vi "App - analyze RUS V6.vi"() -> ()   [LabVIEW 2021] (continued)
"last mod"=timestamp(3493848079 s since 1904-01-01), "file name str"="D:\\Data\\Ultrasound\\LSCO\\LSCO22__130814c\\5_Cooling_2nd_try\\September_2014\\091714\\14.95900K_500_2500_2.10000V_0.00000T_Sep17-2014__21-21-19_001_091714.bin", "mod time(min)"=58230801.31666667, "file format"=enum."binary", "power(V)"=2.1, "Magn Field(T) "=0.0}, {"temperature"=14.952, "temperature str"="14.95200", "file path"=path "D:/Data/Ultrasound/LSCO/LSCO22__130814c/5_Cooling_2nd_try/September_2014/091714/14.95200K_500_2500_2.10000V_0.00000T_Sep17-2014__21-22-38_001_091714.bin", "last mod"=timestamp(3493848158 s since 1904-01-01), "file name str"="D:\\Data\\Ultrasound\\LSCO\\LSCO22__130814c\\5_Cooling_2nd_try\\September_2014\\091714\\14.95200K_500_2500_2.10000V_0.00000T_Sep17-2014__21-22-38_001_091714.bin", "mod time(min)"=58230802.63333333, "file format"=enum."binary", "power(V)"=2.1, "Magn Field(T) "=0.0}, {"temperature"=14.954, "temperature str"="14.95400", "file path"=path "D:/Data/Ultrasound/LSCO/LSCO22__130814c/5_Cooling_2nd_try/September_2014/091714/14.95400K_500_2500_2.10000V_0.00000T_Sep17-2014__21-23-58_001_091714.bin", "last mod"=timestamp(3493848238 s since 1904-01-01), "file name str"="D:\\Data\\Ultrasound\\LSCO\\LSCO22__130814c\\5_Cooling_2nd_try\\September_2014\\091714\\14.95400K_500_2500_2.10000V_0.00000T_Sep17-2014__21-23-58_001_091714.bin", "mod time(min)"=58230803.96666667, "file format"=enum."binary", "power(V)"=2.1, "Magn Field(T) "=0.0}, {"temperature"=14.948, "temperature str"="14.94800", "file path"=path "D:/Data/Ultrasound/LSCO/LSCO22__130814c/5_Cooling_2nd_try/September_2014/091714/14.94800K_500_2500_2.10000V_0.00000T_Sep17-2014__21-25-17_001_091714.bin", "last mod"=timestamp(3493848317 s since 1904-01-01), "file name str"="D:\\Data\\Ultrasound\\LSCO\\LSCO22__130814c\\5_Cooling_2nd_try\\September_2014\\091714\\14.94800K_500_2500_2.10000V_0.00000T_Sep17-2014__21-25-17_001_091714.bin", "mod time(min)"=58230805.28333333, "file format"=enum."binary", "power(V)"=2.1, "Magn Field(T) "=0.0}, {"temperature"=14.938, "temperature str"="14.93800", "file path"=path "D:/Data/Ultrasound/LSCO/LSCO22__130814c/5_Cooling_2nd_try/September_2014/091714/14.93800K_500_2500_2.10000V_0.00000T_Sep17-2014__21-26-37_001_091714.bin", "last mod"=timestamp(3493848397 s since 1904-01-01), "file name str"="D:\\Data\\Ultrasound\\LSCO\\LSCO22__130814c\\5_Cooling_2nd_try\\September_2014\\091714\\14.93800K_500_2500_2.10000V_0.00000T_Sep17-2014__21-26-37_001_091714.bin", "mod time(min)"=58230806.61666667, "file format"=enum."binary", "power(V)"=2.1, "Magn Field(T) "=0.0}, {"temperature"=14.942, "temperature str"="14.94200", "file path"=path "D:/Data/Ultrasound/LSCO/LSCO22__130814c/5_Cooling_2nd_try/September_2014/091714/14.94200K_500_2500_2.10000V_0.00000T_Sep17-2014__21-27-56_001_091714.bin", "last mod"=timestamp(3493848476 s since 1904-01-01), "file name str"="D:\\Data\\Ultrasound\\LSCO\\LSCO22__130814c\\5_Cooling_2nd_try\\September_2014\\091714\\14.94200K_500_2500_2.10000V_0.00000T_Sep17-2014__21-27-56_001_091714.bin", "mod time(min)"=58230807.93333333, "file format"=enum."binary", "power(V)"=2.1, "Magn Field(T) "=0.0}, {"temperature"=14.929, "temperature str"="14.92900", "file path"=path "D:/Data/Ultrasound/LSCO/LSCO22__130814c/5_Cooling_2nd_try/September_2014/091714/14.92900K_500_2500_2.10000V_0.00000T_Sep17-2014__21-29-15_001_091714.bin", "last mod"=timestamp(3493848555 s since 1904-01-01), "file name str"="D:\\Data\\Ultrasound\\LSCO\\LSCO22__130814c\\5_Cooling_2nd_try\\September_2014\\091714\\14.92900K_500_2500_2.10000V_0.00000T_Sep17-2014__21-29-15_001_091714.bin", "mod time(min)"=58230809.25, "file format"=enum."binary", "power(V)"=2.1, "Magn Field(T) "=0.0}, {"temperature"=14.927, "temperature str"="14.92700", "file path"=path "D:/Data/Ultrasound/LSCO/LSCO22__130814c/5_Cooling_2nd_try/September_2014/091714/14.92700K_500_2500_2.10000V_0.00000T_Sep17-2014__21-30-35_001_091714.bin", "last mod"=timestamp(3493848635 s since 1904-01-01), "file name str"="D:\\Data\\Ultrasound\\LSCO\\LSCO22__130814c\\5_Cooling_2nd_try\\September_2014\\091714\\14.92700K_500_2500_2.10000V_0.00000T_Sep17-2014__21-30-35_001_091714.bin", "mod time(min)"=58230810.583333336, "file format"=enum."binary", "power(V)"=2.1, "Magn Field(T) "=0.0}, {"temperature"=14.922, "temperature str"="14.92200", "file path"=path "D:/Data/Ultrasound/LSCO/LSCO22__130814c/5_Cooling_2nd_try/September_2014/091714/14.92200K_500_2500_2.10000V_0.00000T_Sep17-2014__21-31-54_001_091714.bin", "last mod"=timestamp(3493848714 s since 1904-01-01), "file name str"="D:\\Data\\Ultrasound\\LSCO\\LSCO22__130814c\\5_Cooling_2nd_try\\September_2014\\091714\\14.92200K_500_2500_2.10000V_0.00000T_Sep17-2014__21-31-54_001_091714.bin", "mod time(min)"=58230811.9, "file format"=enum."binary", "power(V)"=2.1, "Magn Field(T) "=0.0}, {"temperature"=14.929, "temperature str"="14.92900", "file path"=path "D:/Data/Ultrasound/LSCO/LSCO22__130814c/5_Cooling_2nd_try/September_2014/091714/14.92900K_500_2500_2.10000V_0.00000T_Sep17-2014__21-33-14_001_091714.bin", "last mod"=timestamp(3493848794 s since 1904-01-01), "file name str"="D:\\Data\\Ultrasound\\LSCO\\LSCO22__130814c\\5_Cooling_2nd_try\\September_2014\\091714\\14.92900K_500_2500_2.10000V_0.00000T_Sep17-2014__21-33-14_001_091714.bin", "mod time(min)"=58230813.233333334, "file format"=enum."binary", "power(V)"=2.1, "Magn Field(T) "=0.0}, {"temperature"=14.927, "temperature str"="14.92700", "file path"=path "D:/Data/Ultrasound/LSCO/LSCO22__130814c/5_Cooling_2nd_try/September_2014/091714/14.92700K_500_2500_2.10000V_0.00000T_Sep17-2014__21-34-33_001_091714.bin", "last mod"=timestamp(3493848873 s since 1904-01-01), "file name str"="D:\\Data\\Ultrasound\\LSCO\\LSCO22__130814c\\5_Cooling_2nd_try\\September_2014\\091714\\14.92700K_500_2500_2.10000V_0.00000T_Sep17-2014__21-34-33_001_091714.bin", "mod time(min)"=58230814.55, "file format"=enum."binary", "power(V)"=2.1, "Magn Field(T) "=0.0}, {"temperature"=14.926, "temperature str"="14.92600", "file path"=path "D:/Data/Ultrasound/LSCO/LSCO22__130814c/5_Cooling_2nd_try/September_2014/091714/14.92600K_500_2500_2.10000V_0.00000T_Sep17-2014__21-35-52_001_091714.bin", "last mod"=timestamp(3493848952 s since 1904-01-01), "file name str"="D:\\Data\\Ultrasound\\LSCO\\LSCO22__130814c\\5_Cooling_2nd_try\\September_2014\\091714\\14.92600K_500_2500_2.10000V_0.00000T_Sep17-2014__21-35-52_001_091714.bin", "mod time(min)"=58230815.86666667, "file format"=enum."binary", "power(V)"=2.1, "Magn Field(T) "=0.0}, {"temperature"=14.912, "temperature str"="14.91200", "file path"=path "D:/Data/Ultrasound/LSCO/LSCO22__130814c/5_Cooling_2nd_try/September_2014/091714/14.91200K_500_2500_2.10000V_0.00000T_Sep17-2014__21-37-12_001_091714.bin", "last mod"=timestamp(3493849032 s since 1904-01-01), "file name str"="D:\\Data\\Ultrasound\\LSCO\\LSCO22__130814c\\5_Cooling_2nd_try\\September_2014\\091714\\14.91200K_500_2500_2.10000V_0.00000T_Sep17-2014__21-37-12_001_091714.bin", "mod time(min)"=58230817.2, "file format"=enum."binary", "power(V)"=2.1, "Magn Field(T) "=0.0}, {"temperature"=14.915, "temperature str"="14.91500", "file path"=path "D:/Data/Ultrasound/LSCO/LSCO22__130814c/5_Cooling_2nd_try/September_2014/091714/14.91500K_500_2500_2.10000V_0.00000T_Sep17-2014__21-38-31_001_091714.bin", "last mod"=timestamp(3493849111 s since 1904-01-01), "file name str"="D:\\Data\\Ultrasound\\LSCO\\LSCO22__130814c\\5_Cooling_2nd_try\\September_2014\\091714\\14.91500K_500_2500_2.10000V_0.00000T_Sep17-2014__21-38-31_001_091714.bin", "mod time(min)"=58230818.516666666, "file format"=enum."binary", "power(V)"=2.1, "Magn Field(T) "=0.0}, {"temperature"=14.912, "temperature str"="14.91200", "file path"=path "D:/Data/Ultrasound/LSCO/LSCO22__130814c/5_Cooling_2nd_try/September_2014/091714/14.91200K_500_2500_2.10000V_0.00000T_Sep17-2014__21-39-50_001_091714.bin", "last mod"=timestamp(3493849190 s since 1904-01-01), "file name str"="D:\\Data\\Ultrasound\\LSCO\\LSCO22__130814c\\5_Cooling_2nd_try\\September_2014\\091714\\14.91200K_500_2500_2.10000V_0.00000T_Sep17-2014__21-39-50_001_091714.bin", "mod time(min)"=58230819.833333336, "file format"=enum."binary", "power(V)"=2.1, "Magn Field(T) "=0.0}, {"temperature"=14.91, "temperature str"="14.91000", "file path"=path "D:/Data/Ultrasound/LSCO/LSCO22__130814c/5_Cooling_2nd_try/September_2014/091714/14.91000K_500_2500_2.10000V_0.00000T_Sep17-2014__21-41-10_001_091714.bin", "last mod"=timestamp(3493849270 s since 1904-01-01), "file name str"="D:\\Data\\Ultrasound\\LSCO\\LSCO22__130814c\\5_Cooling_2nd_try\\September_2014\\091714\\14.91000K_500_2500_2.10000V_0.00000T_Sep17-2014__21-41-10_001_091714.bin", "mod time(min)"=58230821.166666664, "file format"=enum."binary", "power(V)"=2.1, "Magn Field(T) "=0.0}, {"temperature"=14.907, "temperature str"="14.90700", "file path"=path "D:/Data/Ultrasound/LSCO/LSCO22__130814c/5_Cooling_2nd_try/September_2014/091714/14.90700K_500_2500_2.10000V_0.00000T_Sep17-2014__21-42-29_001_091714.bin", "last mod"=timestamp(3493849349 s since 1904-01-01), "file name str"="D:\\Data\\Ultrasound\\LSCO\\LSCO22__130814c\\5_Cooling_2nd_try\\September_2014\\091714\\14.90700K_500_2500_2.10000V_0.00000T_Sep17-2014__21-42-29_001_091714.bin", "mod time(min)"=58230822.483333334, "file format"=enum."binary", "power(V)"=2.1, "Magn Field(T) "=0.0}, {"temperature"=14.908, "temperature str"="14.90800", "file path"=path "D:/Data/Ultrasound/LSCO/LSCO22__130814c/5_Cooling_2nd_try/September_2014/091714/14.90800K_500_2500_2.10000V_0.00000T_Sep17-2014__21-43-49_001_091714.bin", "last mod"=timestamp(3493849429 s since 1904-01-01), "file name str"="D:\\Data\\Ultrasound\\LSCO\\LSCO22__130814c\\5_Cooling_2nd_try\\September_2014\\091714\\14.90800K_500_2500_2.10000V_0.00000T_Sep17-2014__21-43-49_001_091714.bin", "mod time(min)"=58230823.81666667, "file format"=enum."binary", "power(V)"=2.1, "Magn Field(T) "=0.0}, {"temperature"=14.9, "temperature str"="14.90000", "file path"=path "D:/Data/Ultrasound/LSCO/LSCO22__130814c/5_Cooling_2nd_try/September_2014/091714/14.90000K_500_2500_2.10000V_0.00000T_Sep17-2014__21-45-08_001_091714.bin", "last mod"=timestamp(3493849508 s since 1904-01-01), "file name str"="D:\\Data\\Ultrasound\\LSCO\\LSCO22__130814c\\5_Cooling_2nd_try\\September_2014\\091714\\14.90000K_500_2500_2.10000V_0.00000T_Sep17-2014__21-45-08_001_091714.bin", "mod time(min)"=58230825.13333333, "file format"=enum."binary", "power(V)"=2.1, "Magn Field(T) "=0.0}, {"temperature"=14.9, "temperature str"="14.90000", "file path"=path "D:/Data/Ultrasound/LSCO/LSCO22__130814c/5_Cooling_2nd_try/September_2014/091714/14.90000K_500_2500_2.10000V_0.00000T_Sep17-2014__21-46-27_001_091714.bin", "last mod"=timestamp(3493849587 s since 1904-01-01), "file name str"="D:\\Data\\Ultrasound\\LSCO\\LSCO22__130814c\\5_Cooling_2nd_try\\September_2014\\091714\\14.90000K_500_2500_2.10000V_0.00000T_Sep17-2014__21-46-27_001_091714.bin", "mod time(min)"=58230826.45, "file format"=enum."binary", "power(V)"=2.1, "Magn Field(T) "=0.0}, {"temperature"=14.895, "temperature str"="14.89500", "file path"=path "D:/Data/Ultrasound/LSCO/LSCO22__130814c/5_Cooling_2nd_try/September_2014/091714/14.89500K_500_2500_2.10000V_0.00000T_Sep17-2014__21-47-47_001_091714.bin", "last mod"=timestamp(3493849667 s since 1904-01-01), "file name str"="D:\\Data\\Ultrasound\\LSCO\\LSCO22__130814c\\5_Cooling_2nd_try\\September_2014\\091714\\14.89500K_500_2500_2.10000V_0.00000T_Sep17-2014__21-47-47_001_091714.bin", "mod time(min)"=58230827.78333333, "file format"=enum."binary", "power(V)"=2.1, "Magn Field(T) "=0.0}, {"temperature"=14.89, "temperature str"="14.89000", "file path"=path "D:/Data/Ultrasound/LSCO/LSCO22__130814c/5_Cooling_2nd_try/September_2014/091714/14.89000K_500_2500_2.10000V_0.00000T_Sep17-2014__21-49-06_001_091714.bin", "last mod"=timestamp(3493849746 s since 1904-01-01), "file name str"="D:\\Data\\Ultrasound\\LSCO\\LSCO22__130814c\\5_Cooling_2nd_try\\September_2014\\091714\\14.89000K_500_2500_2.10000V_0.00000T_Sep17-2014__21-49-06_001_091714.bin", "mod time(min)"=58230829.1, "file format"=enum."binary", "power(V)"=2.1, "Magn Field(T) "=0.0}, {"temperature"=14.886, "temperature str"="14.88600", "file path"=path "D:/Data/Ultrasound/LSCO/LSCO22__130814c/5_Cooling_2nd_try/September_2014/091714/14.88600K_500_2500_2.10000V_0.00000T_Sep17-2014__21-50-26_001_091714.bin", "last mod"=timestamp(3493849826 s since 1904-01-01), "file name str"="D:\\Data\\Ultrasound\\LSCO\\LSCO22__130814c\\5_Cooling_2nd_try\\September_2014\\091714\\14.88600K_500_2500_2.10000V_0.00000T_Sep17-2014__21-50-26_001_091714.bin", "mod time(min)"=58230830.43333333, "file format"=enum."binary", "power(V)"=2.1, "Magn Field(T) "=0.0}, {"temperature"=14.883, "temperature str"="14.88300", "file path"=path "D:/Data/Ultrasound/LSCO/LSCO22__130814c/5_Cooling_2nd_try/September_2014/091714/14.88300K_500_2500_2.10000V_0.00000T_Sep17-2014__21-51-45_001_091714.bin", "last mod"=timestamp(3493849905 s since 1904-01-01), "file name str"="D:\\Data\\Ultrasound\\LSCO\\LSCO22__130814c\\5_Cooling_2nd_try\\September_2014\\091714\\14.88300K_500_2500_2.10000V_0.00000T_Sep17-2014__21-51-45_001_091714.bin", "mod time(min)"=58230831.75, "file format"=enum."binary", "power(V)"=2.1, "Magn Field(T) "=0.0}, {"temperature"=14.876, "temperature str"="14.87600", "file path"=path "D:/Data/Ultrasound/LSCO/LSCO22__130814c/5_Cooling_2nd_try/September_2014/091714/14.87600K_500_2500_2.10000V_0.00000T_Sep17-2014__21-53-04_001_091714.bin", "last mod"=timestamp(3493849984 s since 1904-01-01), "file name str"="D:\\Data\\Ultrasound\\LSCO\\LSCO22__130814c\\5_Cooling_2nd_try\\September_2014\\091714\\14.87600K_500_2500_2.10000V_0.00000T_Sep17-2014__21-53-04_001_091714.bin", "mod time(min)"=58230833.06666667, "file format"=enum."binary", "power(V)"=2.1, "Magn Field(T) "=0.0}, {"temperature"=14.875, "temperature str"="14.87500", "file path"=path "D:/Data/Ultrasound/LSCO/LSCO22__130814c/5_Cooling_2nd_try/September_2014/091714/14.87500K_500_2500_2.10000V_0.00000T_Sep17-2014__21-54-24_001_091714.bin", "last mod"=timestamp(3493850064 s since 1904-01-01), "file name str"="D:\\Data\\Ultrasound\\LSCO\\LSCO22__130814c\\5_Cooling_2nd_try\\September_2014\\091714\\14.87500K_500_2500_2.10000V_0.00000T_Sep17-2014__21-54-24_001_091714.bin", "mod time(min)"=58230834.4, "file format"=enum."binary", "power(V)"=2.1, "Magn Field(T) "=0.0}, {"temperature"=14.872, "temperature str"="14.87200", "file path"=path "D:/Data/Ultrasound/LSCO/LSCO22__130814c/5_Cooling_2nd_try/September_2014/091714/14.87200K_500_2500_2.10000V_0.00000T_Sep17-2014__21-55-43_001_091714.bin", "last mod"=timestamp(3493850143 s since 1904-01-01), "file name str"="D:\\Data\\Ultrasound\\LSCO\\LSCO22__130814c\\5_Cooling_2nd_try\\September_2014\\091714\\14.87200K_500_2500_2.10000V_0.00000T_Sep17-2014__21-55-43_001_091714.bin", "mod time(min)"=58230835.71666667, "file format"=enum."binary", "power(V)"=2.1, "Magn Field(T) "=0.0}, {"temperature"=14.874, "temperature str"="14.87400", "file path"=path "D:/Data/Ultrasound/LSCO/LSCO22__130814c/5_Cooling_2nd_try/September_2014/091714/14.87400K_500_2500_2.10000V_0.00000T_Sep17-2014__21-57-02_001_091714.bin", "last mod"=timestamp(3493850222 s since 1904-01-01), "file name str"="D:\\Data\\Ultrasound\\LSCO\\LSCO22__130814c\\5_Cooling_2nd_try\\September_2014\\091714\\14.87400K_500_2500_2.10000V_0.00000T_Sep17-2014__21-57-02_001_091714.bin", "mod time(min)"=58230837.03333333, "file format"=enum."binary", "power(V)"=2.1, "Magn Field(T) "=0.0}, {"temperature"=14.877, "temperature str"="14.87700", "file path"=path "D:/Data/Ultrasound/LSCO/LSCO22__130814c/5_Cooling_2nd_try/September_2014/091714/14.87700K_500_2500_2.10000V_0.00000T_Sep17-2014__21-58-22_001_091714.bin", "last mod"=timestamp(3493850302 s since 1904-01-01), "file name str"="D:\\Data\\Ultrasound\\LSCO\\LSCO22__130814c\\5_Cooling_2nd_try\\September_2014\\091714\\14.87700K_500_2500_2.10000V_0.00000T_Sep17-2014__21-58-22_001_091714.bin", "mod time(min)"=58230838.36666667, "file format"=enum."binary", "power(V)"=2.1, "Magn Field(T) "=0.0}, {"temperature"=14.872, "temperature str"="14.87200", "file path"=path "D:/Data/Ultrasound/LSCO/LSCO22__130814c/5_Cooling_2nd_try/September_2014/091714/14.87200K_500_2500_2.10000V_0.00000T_Sep17-2014__21-59-41_001_091714.bin", "last mod"=timestamp(3493850381 s since 1904-01-01), "file name str"="D:\\Data\\Ultrasound\\LSCO\\LSCO22__130814c\\5_Cooling_2nd_try\\September_2014\\091714\\14.87200K_500_2500_2.10000V_0.00000T_Sep17-2014__21-59-41_001_091714.bin", "mod time(min)"=58230839.68333333, "file format"=enum."binary", "power(V)"=2.1, "Magn Field(T) "=0.0}, {"temperature"=14.873, "temperature str"="14.87300", "file path"=path "D:/Data/Ultrasound/LSCO/LSCO22__130814c/5_Cooling_2nd_try/September_2014/091714/14.87300K_500_2500_2.10000V_0.00000T_Sep17-2014__22-01-01_001_091714.bin", "last mod"=timestamp(3493850461 s since 1904-01-01), "file name str"="D:\\Data\\Ultrasound\\LSCO\\LSCO22__130814c\\5_Cooling_2nd_try\\September_2014\\091714\\14.87300K_500_2500_2.10000V_0.00000T_Sep17-2014__22-01-01_001_091714.bin", "mod time(min)"=58230841.016666666, "file format"=enum."binary", "power(V)"=2.1, "Magn Field(T) "=0.0}, {"temperature"=14.873, "temperature str"="14.87300", "file path"=path "D:/Data/Ultrasound/LSCO/LSCO22__130814c/5_Cooling_2nd_try/September_2014/091714/14.87300K_500_2500_2.10000V_0.00000T_Sep17-2014__22-02-20_001_091714.bin", "last mod"=timestamp(3493850540 s since 1904-01-01), "file name str"="D:\\Data\\Ultrasound\\LSCO\\LSCO22__130814c\\5_Cooling_2nd_try\\September_2014\\091714\\14.87300K_500_2500_2.10000V_0.00000T_Sep17-2014__22-02-20_001_091714.bin", "mod time(min)"=58230842.333333336, "file format"=enum."binary", "power(V)"=2.1, "Magn Field(T) "=0.0}, {"temperature"=14.868, "temperature str"="14.86800", "file path"=path "D:/Data/Ultrasound/LSCO/LSCO22__130814c/5_Cooling_2nd_try/September_2014/091714/14.86800K_500_2500_2.10000V_0.00000T_Sep17-2014__22-03-39_001_091714.bin", "last mod"=timestamp(3493850619 s since 1904-01-01), "file name str"="D:\\Data\\Ultrasound\\LSCO\\LSCO22__130814c\\5_Cooling_2nd_try\\September_2014\\091714\\14.86800K_500_2500_2.10000V_0.00000T_Sep17-2014__22-03-39_001_091714.bin", "mod time(min)"=58230843.65, "file format"=enum."binary", "power(V)"=2.1, "Magn Field(T) "=0.0}, {"temperature"=14.859, "temperature str"="14.85900", "file path"=path "D:/Data/Ultrasound/LSCO/LSCO22__130814c/5_Cooling_2nd_try/September_2014/091714/14.85900K_500_2500_2.10000V_0.00000T_Sep17-2014__22-04-59_001_091714.bin", "last mod"=timestamp(3493850699 s since 1904-01-01), "file name str"="D:\\Data\\Ultrasound\\LSCO\\LSCO22__130814c\\5_Cooling_2nd_try\\September_2014\\091714\\14.85900K_500_2500_2.10000V_0.00000T_Sep17-2014__22-04-59_001_091714.bin", "mod time(min)"=58230844.983333334, "file format"=enum."binary", "power(V)"=2.1, "Magn Field(T) "=0.0}, {"temperature"=14.866, "temperature str"="14.86600", "file path"=path "D:/Data/Ultrasound/LSCO/LSCO22__130814c/5_Cooling_2nd_try/September_2014/091714/14.86600K_500_2500_2.10000V_0.00000T_Sep17-2014__22-06-18_001_091714.bin", "last mod"=timestamp(3493850778 s since 1904-01-01), "file name str"="D:\\Data\\Ultrasound\\LSCO\\LSCO22__130814c\\5_Cooling_2nd_try\\September_2014\\091714\\14.86600K_500_2500_2.10000V_0.00000T_Sep17-2014__22-06-18_001_091714.bin", "mod time(min)"=58230846.3, "file format"=enum."binary", "power(V)"=2.1, "Magn Field(T) "=0.0}, {"temperature"=14.858, "temperature str"="14.85800", "file path"=path "D:/Data/Ultrasound/LSCO/LSCO22__130814c/5_Cooling_2nd_try/September_2014/091714/14.85800K_500_2500_2.10000V_0.00000T_Sep17-2014__22-07-37_001_091714.bin", "last mod"=timestamp(3493850857 s since 1904-01-01), "file name str"="D:\\Data\\Ultrasound\\LSCO\\LSCO22__130814c\\5_Cooling_2nd_try\\September_2014\\091714\\14.85800K_500_2500_2.10000V_0.00000T_Sep17-2014__22-07-37_001_091714.bin", "mod time(min)"=58230847.61666667, "file format"=enum."binary", "power(V)"=2.1, "Magn Field(T) "=0.0}, {"temperature"=14.86, "temperature str"="14.86000", "file path"=path "D:/Data/Ultrasound/LSCO/LSCO22__130814c/5_Cooling_2nd_try/September_2014/091714/14.86000K_500_2500_2.10000V_0.00000T_Sep17-2014__22-08-57_001_091714.bin", "last mod"=timestamp(3493850937 s since 1904-01-01), "file name str"="D:\\Data\\Ultrasound\\LSCO\\LSCO22__130814c\\5_Cooling_2nd_try\\September_2014\\091714\\14.86000K_500_2500_2.10000V_0.00000T_Sep17-2014__22-08-57_001_091714.bin", "mod time(min)"=58230848.95, "file format"=enum."binary", "power(V)"=2.1, "Magn Field(T) "=0.0}, {"temperature"=14.866, "temperature str"="14.86600", "file path"=path "D:/Data/Ultrasound/LSCO/LSCO22__130814c/5_Cooling_2nd_try/September_2014/091714/14.86600K_500_2500_2.10000V_0.00000T_Sep17-2014__22-10-16_001_091714.bin", "last mod"=timestamp(3493851016 s since 1904-01-01), "file name str"="D:\\Data\\Ultrasound\\LSCO\\LSCO22__130814c\\5_Cooling_2nd_try\\September_2014\\091714\\14.86600K_500_2500_2.10000V_0.00000T_Sep17-2014__22-10-16_001_091714.bin", "mod time(min)"=58230850.266666666, "file format"=enum."binary", "power(V)"=2.1, "Magn Field(T) "=0.0}, {"temperature"=14.857, "temperature str"="14.85700", "file path"=path "D:/Data/Ultrasound/LSCO/LSCO22__130814c/5_Cooling_2nd_try/September_2014/091714/14.85700K_500_2500_2.10000V_0.00000T_Sep17-2014__22-11-36_001_091714.bin", "last mod"=timestamp(3493851096 s since 1904-01-01), "file name str"="D:\\Data\\Ultrasound\\LSCO\\LSCO22__130814c\\5_Cooling_2nd_try\\September_2014\\091714\\14.85700K_500_2500_2.10000V_0.00000T_Sep17-2014__22-11-36_001_091714.bin", "mod time(min)"=58230851.6, "file format"=enum."binary", "power(V)"=2.1, "Magn Field(T) "=0.0}, {"temperature"=14.853, "temperature str"="14.85300", "file path"=path "D:/Data/Ultrasound/LSCO/LSCO22__130814c/5_Cooling_2nd_try/September_2014/091714/14.85300K_500_2500_2.10000V_0.00000T_Sep17-2014__22-12-55_001_091714.bin", "last mod"=timestamp(3493851175 s since 1904-01-01), "file name str"="D:\\Data\\Ultrasound\\LSCO\\LSCO22__130814c\\5_Cooling_2nd_try\\September_2014\\091714\\14.85300K_500_2500_2.10000V_0.00000T_Sep17-2014__22-12-55_001_091714.bin", "mod time(min)"=58230852.916666664, "file format"=enum."binary", "power(V)"=2.1, "Magn Field(T) "=0.0}, {"temperature"=14.852, "temperature str"="14.85200", "file path"=path "D:/Data/Ultrasound/LSCO/LSCO22__130814c/5_Cooling_2nd_try/September_2014/091714/14.85200K_500_2500_2.10000V_0.00000T_Sep17-2014__22-14-14_001_091714.bin", "last mod"=timestamp(3493851254 s since 1904-01-01), "file name str"="D:\\Data\\Ultrasound\\LSCO\\LSCO22__130814c\\5_Cooling_2nd_try\\September_2014\\091714\\14.85200K_500_2500_2.10000V_0.00000T_Sep17-2014__22-14-14_001_091714.bin", "mod time(min)"=58230854.233333334, "file format"=enum."binary", "power(V)"=2.1, "Magn Field(T) "=0.0}, {"temperature"=14.844, "temperature str"="14.84400", "file path"=path "D:/Data/Ultrasound/LSCO/LSCO22__130814c/5_Cooling_2nd_try/September_2014/091714/14.84400K_500_2500_2.10000V_0.00000T_Sep17-2014__22-15-34_001_091714.bin", "last mod"=timestamp(3493851334 s since 1904-01-01), "file name str"="D:\\Data\\Ultrasound\\LSCO\\LSCO22__130814c\\5_Cooling_2nd_try\\September_2014\\091714\\14.84400K_500_2500_2.10000V_0.00000T_Sep17-2014__22-15-34_001_091714.bin", "mod time(min)"=58230855.56666667, "file format"=enum."binary", "power(V)"=2.1, "Magn Field(T) "=0.0}, {"temperature"=14.841, "temperature str"="14.84100", "file path"=path "D:/Data/Ultrasound/LSCO/LSCO22__130814c/5_Cooling_2nd_try/September_2014/091714/14.84100K_500_2500_2.10000V_0.00000T_Sep17-2014__22-16-53_001_091714.bin", "last mod"=timestamp(3493851413 s since 1904-01-01), "file name str"="D:\\Data\\Ultrasound\\LSCO\\LSCO22__130814c\\5_Cooling_2nd_try\\September_2014\\091714\\14.84100K_500_2500_2.10000V_0.00000T_Sep17-2014__22-16-53_001_091714.bin", "mod time(min)"=58230856.88333333, "file format"=enum."binary", "power(V)"=2.1, "Magn Field(T) "=0.0}, {"temperature"=14.835, "temperature str"="14.83500", "file path"=path "D:/Data/Ultrasound/LSCO/LSCO22__130814c/5_Cooling_2nd_try/September_2014/091714/14.83500K_500_2500_2.10000V_0.00000T_Sep17-2014__22-18-12_001_091714.bin", "last mod"=timestamp(3493851492 s since 1904-01-01), "file name str"="D:\\Data\\Ultrasound\\LSCO\\LSCO22__130814c\\5_Cooling_2nd_try\\September_2014\\091714\\14.83500K_500_2500_2.10000V_0.00000T_Sep17-2014__22-18-12_001_091714.bin", "mod time(min)"=58230858.2, "file format"=enum."binary", "power(V)"=2.1, "Magn Field(T) "=0.0}, {"temperature"=14.822, "temperature str"="14.82200", "file path"=path "D:/Data/Ultrasound/LSCO/LSCO22__130814c/5_Cooling_2nd_try/September_2014/091714/14.82200K_500_2500_2.10000V_0.00000T_Sep17-2014__22-19-32_001_091714.bin", "last mod"=timestamp(3493851572 s since 1904-01-01), "file name str"="D:\\Data\\Ultrasound\\LSCO\\LSCO22__130814c\\5_Cooling_2nd_try\\September_2014\\091714\\14.82200K_500_2500_2.10000V_0.00000T_Sep17-2014__22-19-32_001_091714.bin", "mod time(min)"=58230859.53333333, "file format"=enum."binary", "power(V)"=2.1, "Magn Field(T) "=0.0}, {"temperature"=14.821, "temperature str"="14.82100", "file path"=path "D:/Data/Ultrasound/LSCO/LSCO22__130814c/5_Cooling_2nd_try/September_2014/091714/14.82100K_500_2500_2.10000V_0.00000T_Sep17-2014__22-20-51_001_091714.bin", "last mod"=timestamp(3493851651 s since 1904-01-01), "file name str"="D:\\Data\\Ultrasound\\LSCO\\LSCO22__130814c\\5_Cooling_2nd_try\\September_2014\\091714\\14.82100K_500_2500_2.10000V_0.00000T_Sep17-2014__22-20-51_001_091714.bin", "mod time(min)"=58230860.85, "file format"=enum."binary", "power(V)"=2.1, "Magn Field(T) "=0.0}, {"temperature"=14.824, "temperature str"="14.82400", "file path"=path "D:/Data/Ultrasound/LSCO/LSCO22__130814c/5_Cooling_2nd_try/September_2014/091714/14.82400K_500_2500_2.10000V_0.00000T_Sep17-2014__22-22-11_001_091714.bin", "last mod"=timestamp(3493851731 s since 1904-01-01), "file name str"="D:\\Data\\Ultrasound\\LSCO\\LSCO22__130814c\\5_Cooling_2nd_try\\September_2014\\091714\\14.82400K_500_2500_2.10000V_0.00000T_Sep17-2014__22-22-11_001_091714.bin", "mod time(min)"=58230862.18333333, "file format"=enum."binary", "power(V)"=2.1, "Magn Field(T) "=0.0}, {"temperature"=14.817, "temperature str"="14.81700", "file path"=path "D:/Data/Ultrasound/LSCO/LSCO22__130814c/5_Cooling_2nd_try/September_2014/091714/14.81700K_500_2500_2.10000V_0.00000T_Sep17-2014__22-23-30_001_091714.bin", "last mod"=timestamp(3493851810 s since 1904-01-01), "file name str"="D:\\Data\\Ultrasound\\LSCO\\LSCO22__130814c\\5_Cooling_2nd_try\\September_2014\\091714\\14.81700K_500_2500_2.10000V_0.00000T_Sep17-2014__22-23-30_001_091714.bin", "mod time(min)"=58230863.5, "file format"=enum."binary", "power(V)"=2.1, "Magn Field(T) "=0.0}, {"temperature"=14.811, "temperature str"="14.81100", "file path"=path "D:/Data/Ultrasound/LSCO/LSCO22__130814c/5_Cooling_2nd_try/September_2014/091714/14.81100K_500_2500_2.10000V_0.00000T_Sep17-2014__22-24-49_001_091714.bin", "last mod"=timestamp(3493851889 s since 1904-01-01), "file name str"="D:\\Data\\Ultrasound\\LSCO\\LSCO22__130814c\\5_Cooling_2nd_try\\September_2014\\091714\\14.81100K_500_2500_2.10000V_0.00000T_Sep17-2014__22-24-49_001_091714.bin", "mod time(min)"=58230864.81666667, "file format"=enum."binary", "power(V)"=2.1, "Magn Field(T) "=0.0}, {"temperature"=14.805, "temperature str"="14.80500", "file path"=path "D:/Data/Ultrasound/LSCO/LSCO22__130814c/5_Cooling_2nd_try/September_2014/091714/14.80500K_500_2500_2.10000V_0.00000T_Sep17-2014__22-26-09_001_091714.bin", "last mod"=timestamp(3493851969 s since 1904-01-01), "file name str"="D:\\Data\\Ultrasound\\LSCO\\LSCO22__130814c\\5_Cooling_2nd_try\\September_2014\\091714\\14.80500K_500_2500_2.10000V_0.00000T_Sep17-2014__22-26-09_001_091714.bin", "mod time(min)"=58230866.15, "file format"=enum."binary", "power(V)"=2.1, "Magn Field(T) "=0.0}, {"temperature"=14.791, "temperature str"="14.79100", "file path"=path "D:/Data/Ultrasound/LSCO/LSCO22__130814c/5_Cooling_2nd_try/September_2014/091714/14.79100K_500_2500_2.10000V_0.00000T_Sep17-2014__22-27-28_001_091714.bin", "last mod"=timestamp(3493852048 s since 1904-01-01), "file name str"="D:\\Data\\Ultrasound\\LSCO\\LSCO22__130814c\\5_Cooling_2nd_try\\September_2014\\091714\\14.79100K_500_2500_2.10000V_0.00000T_Sep17-2014__22-27-28_001_091714.bin", "mod time(min)"=58230867.46666667, "file format"=enum."binary", "power(V)"=2.1, "Magn Field(T) "=0.0}, {"temperature"=14.787, "temperature str"="14.78700", "file path"=path "D:/Data/Ultrasound/LSCO/LSCO22__130814c/5_Cooling_2nd_try/September_2014/091714/14.78700K_500_2500_2.10000V_0.00000T_Sep17-2014__22-28-48_001_091714.bin", "last mod"=timestamp(3493852128 s since 1904-01-01), "file name str"="D:\\Data\\Ultrasound\\LSCO\\LSCO22__130814c\\5_Cooling_2nd_try\\September_2014\\091714\\14.78700K_500_2500_2.10000V_0.00000T_Sep17-2014__22-28-48_001_091714.bin", "mod time(min)"=58230868.8, "file format"=enum."binary", "power(V)"=2.1, "Magn Field(T) "=0.0}, {"temperature"=14.778, "temperature str"="14.77800", "file path"=path "D:/Data/Ultrasound/LSCO/LSCO22__130814c/5_Cooling_2nd_try/September_2014/091714/14.77800K_500_2500_2.10000V_0.00000T_Sep17-2014__22-30-07_001_091714.bin", "last mod"=timestamp(3493852207 s since 1904-01-01), "file name str"="D:\\Data\\Ultrasound\\LSCO\\LSCO22__130814c\\5_Cooling_2nd_try\\September_2014\\091714\\14.77800K_500_2500_2.10000V_0.00000T_Sep17-2014__22-30-07_001_091714.bin", "mod time(min)"=58230870.11666667, "file format"=enum."binary", "power(V)"=2.1, "Magn Field(T) "=0.0}, {"temperature"=14.773, "temperature str"="14.77300", "file path"=path "D:/Data/Ultrasound/LSCO/LSCO22__130814c/5_Cooling_2nd_try/September_2014/091714/14.77300K_500_2500_2.10000V_0.00000T_Sep17-2014__22-31-26_001_091714.bin", "last mod"=timestamp(3493852286 s since 1904-01-01), "file name str"="D:\\Data\\Ultrasound\\LSCO\\LSCO22__130814c\\5_Cooling_2nd_try\\September_2014\\091714\\14.77300K_500_2500_2.10000V_0.00000T_Sep17-2014__22-31-26_001_091714.bin", "mod time(min)"=58230871.43333333, "file format"=enum."binary", "power(V)"=2.1, "Magn Field(T) "=0.0}, {"temperature"=14.769, "temperature str"="14.76900", "file path"=path "D:/Data/Ultrasound/LSCO/LSCO22__130814c/5_Cooling_2nd_try/September_2014/091714/14.76900K_500_2500_2.10000V_0.00000T_Sep17-2014__22-32-46_001_091714.bin", "last mod"=timestamp(3493852366 s since 1904-01-01), "file name str"="D:\\Data\\Ultrasound\\LSCO\\LSCO22__130814c\\5_Cooling_2nd_try\\September_2014\\091714\\14.76900K_500_2500_2.10000V_0.00000T_Sep17-2014__22-32-46_001_091714.bin", "mod time(min)"=58230872.766666666, "file format"=enum."binary", "power(V)"=2.1, "Magn Field(T) "=0.0}, {"temperature"=14.763, "temperature str"="14.76300", "file path"=path "D:/Data/Ultrasound/LSCO/LSCO22__130814c/5_Cooling_2nd_try/September_2014/091714/14.76300K_500_2500_2.10000V_0.00000T_Sep17-2014__22-34-05_001_091714.bin", "last mod"=timestamp(3493852445 s since 1904-01-01), "file name str"="D:\\Data\\Ultrasound\\LSCO\\LSCO22__130814c\\5_Cooling_2nd_try\\September_2014\\091714\\14.76300K_500_2500_2.10000V_0.00000T_Sep17-2014__22-34-05_001_091714.bin", "mod time(min)"=58230874.083333336, "file format"=enum."binary", "power(V)"=2.1, "Magn Field(T) "=0.0}, {"temperature"=14.753, "temperature str"="14.75300", "file path"=path "D:/Data/Ultrasound/LSCO/LSCO22__130814c/5_Cooling_2nd_try/September_2014/091714/14.75300K_500_2500_2.10000V_0.00000T_Sep17-2014__22-35-24_001_091714.bin", "last mod"=timestamp(3493852524 s since 1904-01-01), "file name str"="D:\\Data\\Ultrasound\\LSCO\\LSCO22__130814c\\5_Cooling_2nd_try\\September_2014\\091714\\14.75300K_500_2500_2.10000V_0.00000T_Sep17-2014__22-35-24_001_091714.bin", "mod time(min)"=58230875.4, "file format"=enum."binary", "power(V)"=2.1, "Magn Field(T) "=0.0}, {"temperature"=14.749, "temperature str"="14.74900", "file path"=path "D:/Data/Ultrasound/LSCO/LSCO22__130814c/5_Cooling_2nd_try/September_2014/091714/14.74900K_500_2500_2.10000V_0.00000T_Sep17-2014__22-36-44_001_091714.bin", "last mod"=timestamp(3493852604 s since 1904-01-01), "file name str"="D:\\Data\\Ultrasound\\LSCO\\LSCO22__130814c\\5_Cooling_2nd_try\\September_2014\\091714\\14.74900K_500_2500_2.10000V_0.00000T_Sep17-2014__22-36-44_001_091714.bin", "mod time(min)"=58230876.733333334, "file format"=enum."binary", "power(V)"=2.1, "Magn Field(T) "=0.0}, {"temperature"=14.747, "temperature str"="14.74700", "file path"=path "D:/Data/Ultrasound/LSCO/LSCO22__130814c/5_Cooling_2nd_try/September_2014/091714/14.74700K_500_2500_2.10000V_0.00000T_Sep17-2014__22-38-03_001_091714.bin", "last mod"=timestamp(3493852683 s since 1904-01-01), "file name str"="D:\\Data\\Ultrasound\\LSCO\\LSCO22__130814c\\5_Cooling_2nd_try\\September_2014\\091714\\14.74700K_500_2500_2.10000V_0.00000T_Sep17-2014__22-38-03_001_091714.bin", "mod time(min)"=58230878.05, "file format"=enum."binary", "power(V)"=2.1, "Magn Field(T) "=0.0}, {"temperature"=14.742, "temperature str"="14.74200", "file path"=path "D:/Data/Ultrasound/LSCO/LSCO22__130814c/5_Cooling_2nd_try/September_2014/091714/14.74200K_500_2500_2.10000V_0.00000T_Sep17-2014__22-39-23_001_091714.bin", "last mod"=timestamp(3493852763 s since 1904-01-01), "file name str"="D:\\Data\\Ultrasound\\LSCO\\LSCO22__130814c\\5_Cooling_2nd_try\\September_2014\\091714\\14.74200K_500_2500_2.10000V_0.00000T_Sep17-2014__22-39-23_001_091714.bin", "mod time(min)"=58230879.38333333, "file format"=enum."binary", "power(V)"=2.1, "Magn Field(T) "=0.0}, {"temperature"=14.739, "temperature str"="14.73900", "file path"=path "D:/Data/Ultrasound/LSCO/LSCO22__130814c/5_Cooling_2nd_try/September_2014/091714/14.73900K_500_2500_2.10000V_0.00000T_Sep17-2014__22-40-42_001_091714.bin", "last mod"=timestamp(3493852842 s since 1904-01-01), "file name str"="D:\\Data\\Ultrasound\\LSCO\\LSCO22__130814c\\5_Cooling_2nd_try\\September_2014\\091714\\14.73900K_500_2500_2.10000V_0.00000T_Sep17-2014__22-40-42_001_091714.bin", "mod time(min)"=58230880.7, "file format"=enum."binary", "power(V)"=2.1, "Magn Field(T) "=0.0}, {"temperature"=14.735, "temperature str"="14.73500", "file path"=path "D:/Data/Ultrasound/LSCO/LSCO22__130814c/5_Cooling_2nd_try/September_2014/091714/14.73500K_500_2500_2.10000V_0.00000T_Sep17-2014__22-42-01_001_091714.bin", "last mod"=timestamp(3493852921 s since 1904-01-01), "file name str"="D:\\Data\\Ultrasound\\LSCO\\LSCO22__130814c\\5_Cooling_2nd_try\\September_2014\\091714\\14.73500K_500_2500_2.10000V_0.00000T_Sep17-2014__22-42-01_001_091714.bin", "mod time(min)"=58230882.016666666, "file format"=enum."binary", "power(V)"=2.1, "Magn Field(T) "=0.0}, {"temperature"=14.73, "temperature str"="14.73000", "file path"=path "D:/Data/Ultrasound/LSCO/LSCO22__130814c/5_Cooling_2nd_try/September_2014/091714/14.73000K_500_2500_2.10000V_0.00000T_Sep17-2014__22-43-21_001_091714.bin", "last mod"=timestamp(3493853001 s since 1904-01-01), "file name str"="D:\\Data\\Ultrasound\\LSCO\\LSCO22__130814c\\5_Cooling_2nd_try\\September_2014\\091714\\14.73000K_500_2500_2.10000V_0.00000T_Sep17-2014__22-43-21_001_091714.bin", "mod time(min)"=58230883.35, "file format"=enum."binary", "power(V)"=2.1, "Magn Field(T) "=0.0}, {"temperature"=14.731, "temperature str"="14.73100", "file path"=path "D:/Data/Ultrasound/LSCO/LSCO22__130814c/5_Cooling_2nd_try/September_2014/091714/14.73100K_500_2500_2.10000V_0.00000T_Sep17-2014__22-44-40_001_091714.bin", "last mod"=timestamp(3493853080 s since 1904-01-01), "file name str"="D:\\Data\\Ultrasound\\LSCO\\LSCO22__130814c\\5_Cooling_2nd_try\\September_2014\\091714\\14.73100K_500_2500_2.10000V_0.00000T_Sep17-2014__22-44-40_001_091714.bin", "mod time(min)"=58230884.666666664, "file format"=enum."binary", "power(V)"=2.1, "Magn Field(T) "=0.0}, {"temperature"=14.74, "temperature str"="14.74000", "file path"=path "D:/Data/Ultrasound/LSCO/LSCO22__130814c/5_Cooling_2nd_try/September_2014/091714/14.74000K_500_2500_2.10000V_0.00000T_Sep17-2014__22-45-59_001_091714.bin", "last mod"=timestamp(3493853159 s since 1904-01-01), "file name str"="D:\\Data\\Ultrasound\\LSCO\\LSCO22__130814c\\5_Cooling_2nd_try\\September_2014\\091714\\14.74000K_500_2500_2.10000V_0.00000T_Sep17-2014__22-45-59_001_091714.bin", "mod time(min)"=58230885.983333334, "file format"=enum."binary", "power(V)"=2.1, "Magn Field(T) "=0.0}, {"temperature"=14.735, "temperature str"="14.73500", "file path"=path "D:/Data/Ultrasound/LSCO/LSCO22__130814c/5_Cooling_2nd_try/September_2014/091714/14.73500K_500_2500_2.10000V_0.00000T_Sep17-2014__22-47-19_001_091714.bin", "last mod"=timestamp(3493853239 s since 1904-01-01), "file name str"="D:\\Data\\Ultrasound\\LSCO\\LSCO22__130814c\\5_Cooling_2nd_try\\September_2014\\091714\\14.73500K_500_2500_2.10000V_0.00000T_Sep17-2014__22-47-19_001_091714.bin", "mod time(min)"=58230887.31666667, "file format"=enum."binary", "power(V)"=2.1, "Magn Field(T) "=0.0}, {"temperature"=14.742, "temperature str"="14.74200", "file path"=path "D:/Data/Ultrasound/LSCO/LSCO22__130814c/5_Cooling_2nd_try/September_2014/091714/14.74200K_500_2500_2.10000V_0.00000T_Sep17-2014__22-48-38_001_091714.bin", "last mod"=timestamp(3493853318 s since 1904-01-01), "file name str"="D:\\Data\\Ultrasound\\LSCO\\LSCO22__130814c\\5_Cooling_2nd_try\\September_2014\\091714\\14.74200K_500_2500_2.10000V_0.00000T_Sep17-2014__22-48-38_001_091714.bin", "mod time(min)"=58230888.63333333, "file format"=enum."binary", "power(V)"=2.1, "Magn Field(T) "=0.0}, {"temperature"=14.735, "temperature str"="14.73500", "file path"=path "D:/Data/Ultrasound/LSCO/LSCO22__130814c/5_Cooling_2nd_try/September_2014/091714/14.73500K_500_2500_2.10000V_0.00000T_Sep17-2014__22-49-58_001_091714.bin", "last mod"=timestamp(3493853398 s since 1904-01-01), "file name str"="D:\\Data\\Ultrasound\\LSCO\\LSCO22__130814c\\5_Cooling_2nd_try\\September_2014\\091714\\14.73500K_500_2500_2.10000V_0.00000T_Sep17-2014__22-49-58_001_091714.bin", "mod time(min)"=58230889.96666667, "file format"=enum."binary", "power(V)"=2.1, "Magn Field(T) "=0.0}, {"temperature"=14.732, "temperature str"="14.73200", "file path"=path "D:/Data/Ultrasound/LSCO/LSCO22__130814c/5_Cooling_2nd_try/September_2014/091714/14.73200K_500_2500_2.10000V_0.00000T_Sep17-2014__22-51-17_001_091714.bin", "last mod"=timestamp(3493853477 s since 1904-01-01), "file name str"="D:\\Data\\Ultrasound\\LSCO\\LSCO22__130814c\\5_Cooling_2nd_try\\September_2014\\091714\\14.73200K_500_2500_2.10000V_0.00000T_Sep17-2014__22-51-17_001_091714.bin", "mod time(min)"=58230891.28333333, "file format"=enum."binary", "power(V)"=2.1, "Magn Field(T) "=0.0}, {"temperature"=14.732, "temperature str"="14.73200", "file path"=path "D:/Data/Ultrasound/LSCO/LSCO22__130814c/5_Cooling_2nd_try/September_2014/091714/14.73200K_500_2500_2.10000V_0.00000T_Sep17-2014__22-52-36_001_091714.bin", "last mod"=timestamp(3493853556 s since 1904-01-01), "file name str"="D:\\Data\\Ultrasound\\LSCO\\LSCO22__130814c\\5_Cooling_2nd_try\\September_2014\\091714\\14.73200K_500_2500_2.10000V_0.00000T_Sep17-2014__22-52-36_001_091714.bin", "mod time(min)"=58230892.6, "file format"=enum."binary", "power(V)"=2.1, "Magn Field(T) "=0.0}, {"temperature"=14.724, "temperature str"="14.72400", "file path"=path "D:/Data/Ultrasound/LSCO/LSCO22__130814c/5_Cooling_2nd_try/September_2014/091714/14.72400K_500_2500_2.10000V_0.00000T_Sep17-2014__22-53-56_001_091714.bin", "last mod"=timestamp(3493853636 s since 1904-01-01), "file name str"="D:\\Data\\Ultrasound\\LSCO\\LSCO22__130814c\\5_Cooling_2nd_try\\September_2014\\091714\\14.72400K_500_2500_2.10000V_0.00000T_Sep17-2014__22-53-56_001_091714.bin", "mod time(min)"=58230893.93333333, "file format"=enum."binary", "power(V)"=2.1, "Magn Field(T) "=0.0}, {"temperature"=14.722, "temperature str"="14.72200", "file path"=path "D:/Data/Ultrasound/LSCO/LSCO22__130814c/5_Cooling_2nd_try/September_2014/091714/14.72200K_500_2500_2.10000V_0.00000T_Sep17-2014__22-55-15_001_091714.bin", "last mod"=timestamp(3493853715 s since 1904-01-01), "file name str"="D:\\Data\\Ultrasound\\LSCO\\LSCO22__130814c\\5_Cooling_2nd_try\\September_2014\\091714\\14.72200K_500_2500_2.10000V_0.00000T_Sep17-2014__22-55-15_001_091714.bin", "mod time(min)"=58230895.25, "file format"=enum."binary", "power(V)"=2.1, 
